vi "tmp_toml_load.vi"(4 "vi":refnum<vi>, 8 "error in (no error)":errorcluster, 10 "operation (open or create)":T1(ring)=enum."open or create", 11 "path in":path) -> (0 "error out":errorcluster, 2 "file exists":bool, 3 "path out":path)   [LabVIEW 2017]
uses:
  <vilib>/Utility/error.llb/Clear Errors.vi
  <vilib>/Utility/file.llb/Application Directory.vi
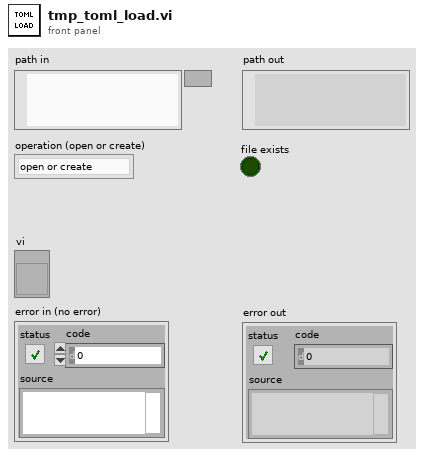
[diagram p1: front panel]
types:
  T1 = enum16{"open", "replace", "create", "open or create", "replace or create", "replace or create with confirmation"}
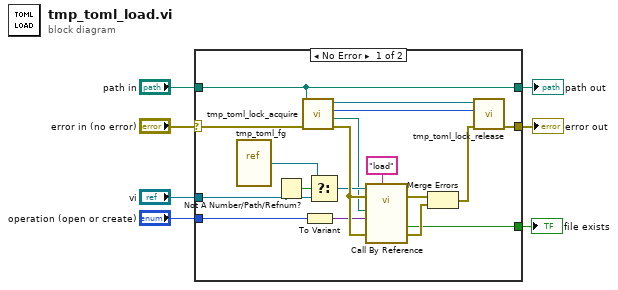
[diagram p0: block diagram]
diagram:
  n1 = case shown="No Error" "error in (no error)" {
    selector: "error in (no error)" -> [w23 w26]
    tunnel: [w19 w26] -> w6
    tunnel: "vi" -> [w16 _]
    tunnel: "path in" -> [w13 w27]
    tunnel: [w13 w27] -> w3
    tunnel: "operation (open or create)" -> [w9 _]
    tunnel: [w10 _] -> w1
    frame No Error {
      n2 = vi-ref "tmp_toml_fg.vi"() -> (w15:refnum<vi>)
      n3 = Not A Number/Path/Refnum?(number/path/refnum=w16) -> (NaN/Path/Refnum?=w17:bool)
      n4 = call "tmp_toml_lock_acquire.vi"("error in (no error)"=w23, "path in"=w13) -> ("error out"=w22:errorcluster, "resolved path"=w12:path, "cnt"=w24:u8, "lock"=w25:refnum<queue>)  [unwired: 6 in]
      n5 = To Variant(anything=w9) -> (Variant=w8:variant)
      n6 = Select(t=w15, s=w17, f=w16) -> (s? t:f=w14:refnum<vi>)
      n7 = call-by-ref "?"(reference=w14, error in=w22, "cmd"="load", 8:"error in (no error)"=w22, "data in"=w8, "path in"=w12) -> (error out=w21:errorcluster, 0:"error out"=w11:errorcluster, "return"=w10:bool)  [unwired: 4 in, 3 out]
      n8 = Merge Errors(w21, w11) -> (w20:errorcluster)
      n9 = call "tmp_toml_lock_release.vi"("error in (no error)"=w20, "cnt"=w24, "lock"=w25) -> ("error out"=w19:errorcluster)  [unwired: 8 in]
    }
    frame Error {
    }
  }
  "error out" <- w6
  "path out" <- w3
  "file exists" <- w1
